vi "LL Sensor Fusion.vi"() -> ()   [LabVIEW 2019]
uses:
  <vilib>/Rock Robotics/Network Tables/NT Read Number.vi
panel:
  in  "Estimated Heading to Target (deg)":dbl
  in  "Robot H (deg)":dbl
  in  "LimeLight Valid":bool
  out "Fused Heading to Target":dbl
  in  "loop cycles to average":i32=15
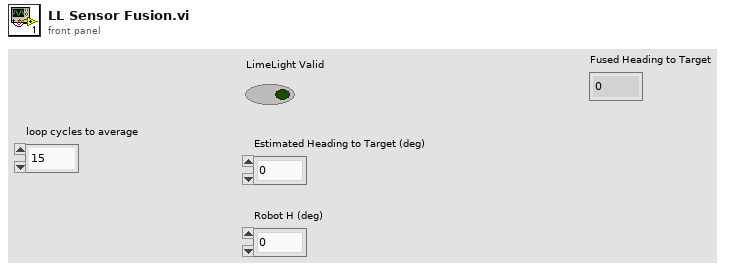
[diagram p1: front panel]
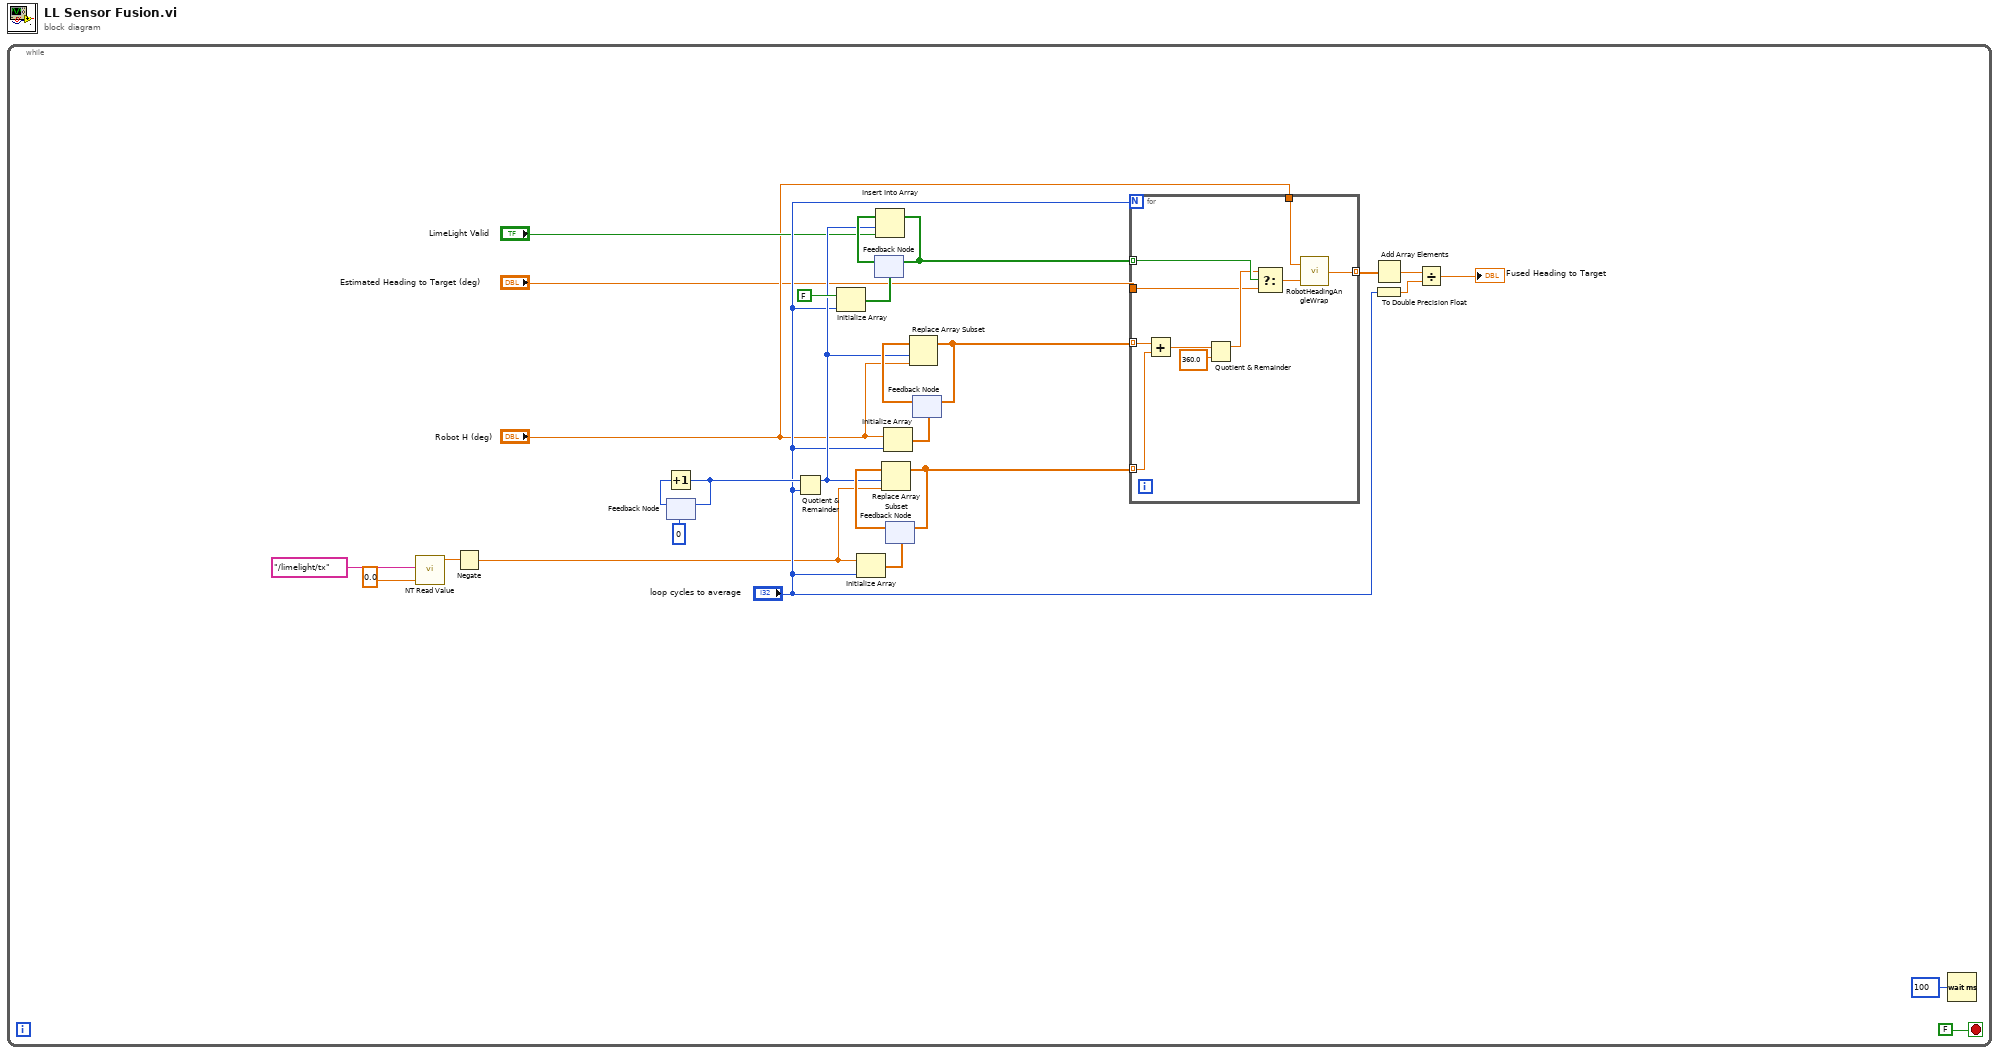
[diagram p0: block diagram]
diagram:
  n1 = while {
    stop <- FALSE stop-if-true
    n2 = call-poly <vilib>:"NT Read Value.vi"("Default Value"=0.0, "Name"="/limelight/tx") -> ("Numeric"=w26:dbl)  [unwired: 8 in, 1 out]
    n3 = Negate(x=w26) -> (-x=w7:dbl)
    n4 = feedback #1(0) -> (w22:i32)
    n5 = Increment(x=w22) -> (x+1=w21:i32)
    n6 = feedback-in #1(w21) -> ()
    n7 = Quotient & Remainder(x=w21, y="loop cycles to average") -> (x-y*floor(x/y)=w13:i32)  [unwired: 1 out]
    n8 = Initialize Array(FALSE, "loop cycles to average") -> (w18:bool[])
    n9 = Initialize Array(w7, "loop cycles to average") -> (w25:dbl[])
    n10 = feedback #2(w18) -> (w20:bool[])
    n11 = Insert Into Array(array=w20, index=w13, new element="LimeLight Valid") -> (w17:bool[])
    n12 = feedback-in #2(w17) -> ()
    n13 = Initialize Array("Robot H (deg)", "loop cycles to average") -> (w15:dbl[])
    n14 = feedback #3(w25) -> (w24:dbl[])
    n15 = Replace Array Subset(array=w24, new element=w7, index=w13) -> (w16:dbl[])
    n16 = feedback-in #3(w16) -> ()
    n17 = feedback #4(w15) -> (w14:dbl[])
    n18 = Replace Array Subset(array=w14, new element="Robot H (deg)", index=w13) -> (w12:dbl[])
    n19 = feedback-in #4(w12) -> ()
    n20 = for {
      N: "loop cycles to average" -> [_]
      tunnel: w17 -> [w38] mode=indexing
      tunnel: w16 -> [w35] mode=indexing
      tunnel: "Estimated Heading to Target (deg)" -> [w33]
      tunnel: w12 -> [w32] mode=indexing
      tunnel: "Robot H (deg)" -> [w31]
      tunnel: [w29] -> w11 mode=indexing
      n21 = Add(x=w32, y=w35) -> (x+y=w37:dbl)
      n22 = Quotient & Remainder(x=w37, y=360.0) -> (x-y*floor(x/y)=w34:dbl)  [unwired: 1 out]
      n23 = Select(t=w34, s=w38, f=w33) -> (s? t:f=w30:dbl)
      n24 = call "RobotHeadingAngleWrap.vi"("Goal Angle (deg)"=w30, "Current Angle (deg)"=w31) -> ("Angular Distance (deg)"=w29:dbl)
    }
    n25 = Add Array Elements(numeric array=w11) -> (sum=w10:dbl)
    n26 = To Double Precision Float(number="loop cycles to average") -> (double precision float=w9:dbl)
    n27 = Divide(x=w10, y=w9) -> (x/y=→"Fused Heading to Target":dbl)
    n28 = Wait (ms)(milliseconds to wait=u32 100) -> ()  [unwired: 1 out]
  }
